vi "Write connections.vi"(8 "error in (no error)":errorcluster, 10 "Baseline-Mocon piD-TECH plus":T1, 11 "Baseline Mocon piD-Tech plus in":refnum<class "Baseline Mocon piD-Tech plus.lvclass">) -> (0 "error out":errorcluster, 3 "Baseline Mocon piD-Tech plus out":refnum<class "Baseline Mocon piD-Tech plus.lvclass">)   [LabVIEW 2011, in "Baseline Mocon piD-Tech plus.lvclass"]
uses:
  Baseline Mocon piD-Tech plus.lvclass
  Connections.ctl
  Baseline Mocon piD-Tech plus.lvclass/Baseline Mocon piD-Tech plus.ctl
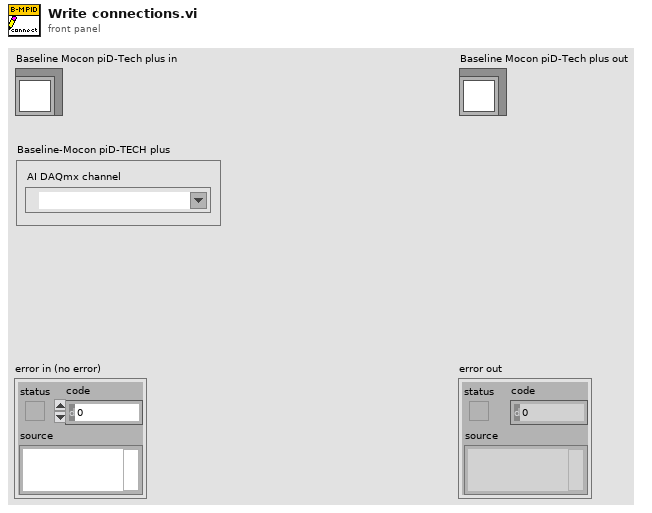
[diagram p1: front panel]
types:
  T1 = typedef "Baseline Mocon piD-Tech plus.lvclass/Connections.ctl" = cluster{"AI DAQmx channel":tag}
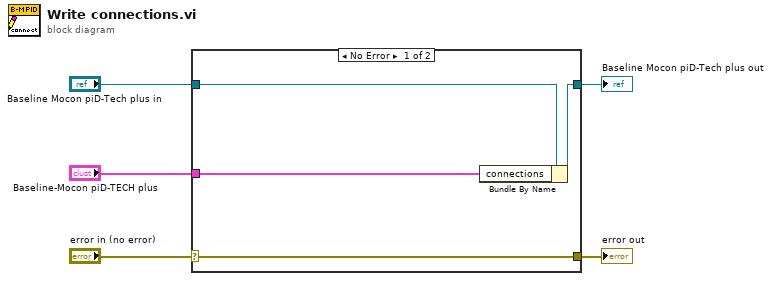
[diagram p0: block diagram]
diagram:
  n1 = case shown="No Error" "error in (no error)" {
    selector: "error in (no error)" -> [w9 w10]
    tunnel: [w9 w10] -> w4
    tunnel: [w7 w11] -> w2
    tunnel: "Baseline Mocon piD-Tech plus in" -> [w8 w11]
    tunnel: "Baseline-Mocon piD-TECH plus" -> [w6 _]
    frame No Error {
      n2 = Bundle By Name(cluster=w8, "connections"=w6) -> (w7:refnum<class "Baseline Mocon piD-Tech plus.lvclass">)
    }
    frame Error {
    }
  }
  "error out" <- w4
  "Baseline Mocon piD-Tech plus out" <- w2
